vi "SparseCoder.vi"(8 "error in":errorcluster) -> (0 "error out":errorcluster, 3 "out":refnum<class "SparseCoder.lvclass">)   [LabVIEW 2020]
doc: "Sparse coding\n\n Finds a sparse representation of data against a fixed, precomputed\n dictionary.\n\n Each row of the result is the solution to a sparse coding problem.\n The goal is to find a sparse array `code` such that::\n\n X ~= code * dictionary\n\n Read more in the :ref:`User Guide <SparseCoder>`.\n\n Parameters\n ----------\n dictionary : ndarray of shape (n_components, n_features)\n The dictionary atoms used for sparse coding. Lines are assumed to be\n normalized to unit norm.\n\n transform_algorithm : {'lasso_lars', 'lasso_cd', 'lars', 'omp', 'threshold'}, default='omp'\n Algorithm used to transform the data:\n\n - `'lars'`: uses the least angle regression method\n (`linear_model.lars_path`);\n - `'lasso_lars'`: uses Lars to compute the Lasso solution;\n - `'lasso_cd'`: uses the coordinate descent method to compute the\n Lasso solution (linear_model.Lasso). `'lasso_lars'` will be faster if\n the estimated components are sparse;\n - `'omp'`: uses orthogonal matching pursuit to estimate the sparse\n solution;\n - `'threshold'`: squashes to zero all coefficients less than alpha from\n the projection ``dictionary * X'``.\n\n transform_n_nonzero_coefs : int, default=None\n Number of nonzero coefficients to target in each column of the\n solution. This is only used by `algorithm='lars'` and `algorithm='omp'`\n and is overridden by `alpha` in the `omp` case. If `None`, then\n `transform_n_nonzero_coefs=int(n_features / 10)`.\n\n transform_alpha : float, default=None\n If `algorithm='lasso_lars'` or `algorithm='lasso_cd'`, `alpha` is the\n penalty applied to the L1 norm.\n If `algorithm='threshold'`, `alpha` is the absolute value of the\n threshold below which coefficients will be squashed to zero.\n If `algorithm='omp'`, `alpha` is the tolerance parameter: the value of\n the reconstruction error targeted. In this case, it overrides\n `n_nonzero_coefs`.\n If `None`, default to 1.\n\n split_sign : bool, default=False\n Whether to split the sparse feature vector into the concatenation of\n its negative part and its positive part. This can improve the\n performance of downstream classifiers.\n\n n_jobs : int, default=None\n Number of parallel jobs to run.\n ``None`` means 1 unless in a :obj:`joblib.parallel_backend` context.\n ``-1`` means using all processors. See :term:`Glossary <n_jobs>`\n for more details.\n\n positive_code : bool, default=False\n Whether to enforce positivity when finding the code.\n\n .. versionadded:: 0.20\n\n transform_max_iter : int, default=1000\n Maximum number of iterations to perform if `algorithm='lasso_cd'` or\n `lasso_lars`.\n\n .. versionadded:: 0.22\n\n Attributes\n ----------\n components_ : ndarray of shape (n_components, n_features)\n The unchanged dictionary atoms.\n\n .. deprecated:: 0.24\n This attribute is deprecated in 0.24 and will be removed in\n 1.1 (renaming of 0.26). Use `dictionary` instead.\n\n \nAvailable methods:\nFit\nFit Transform\nTransform\nGet Attributes\nGet Params\nSet Params"
uses:
  SparseCoder.lvclass
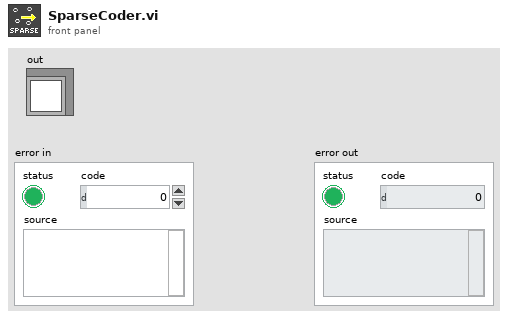
[diagram p1: front panel]
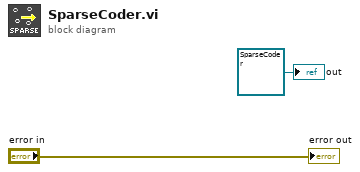
[diagram p0: block diagram]
diagram:
  "out" <- refnum<class "SparseCoder.lvclass"> refnum ("model")
  "error out" <- "error in"
